vi "extract group name.vi"(9 "dictionary":T1, 10 "supported types":T2[](array[typedef]), 11 "TDMS datalogger configuration in":refnum<class "TDMS datalogger configuration.lvclass">) -> (2 "dictionary group names":T1)   [LabVIEW 2015, in "TDMS datalogger runtime.lvclass"]
uses:
  TDMS datalogger runtime.lvclass
  <vilib>/NI/Tag Bus/dictionary/full data dictionary.ctl
  <vilib>/NI/Tag Bus/tag/Data Type.ctl
  configuration/TDMS datalogger configuration.lvclass
  <vilib>/NI/Tag Bus/tag/tag descriptor.lvclass/tag descriptor.ctl
  <vilib>/NI/Tag Bus/tag/tag descriptor.lvclass
  <vilib>/NI/Tag Bus/dictionary/data dictionary.lvclass
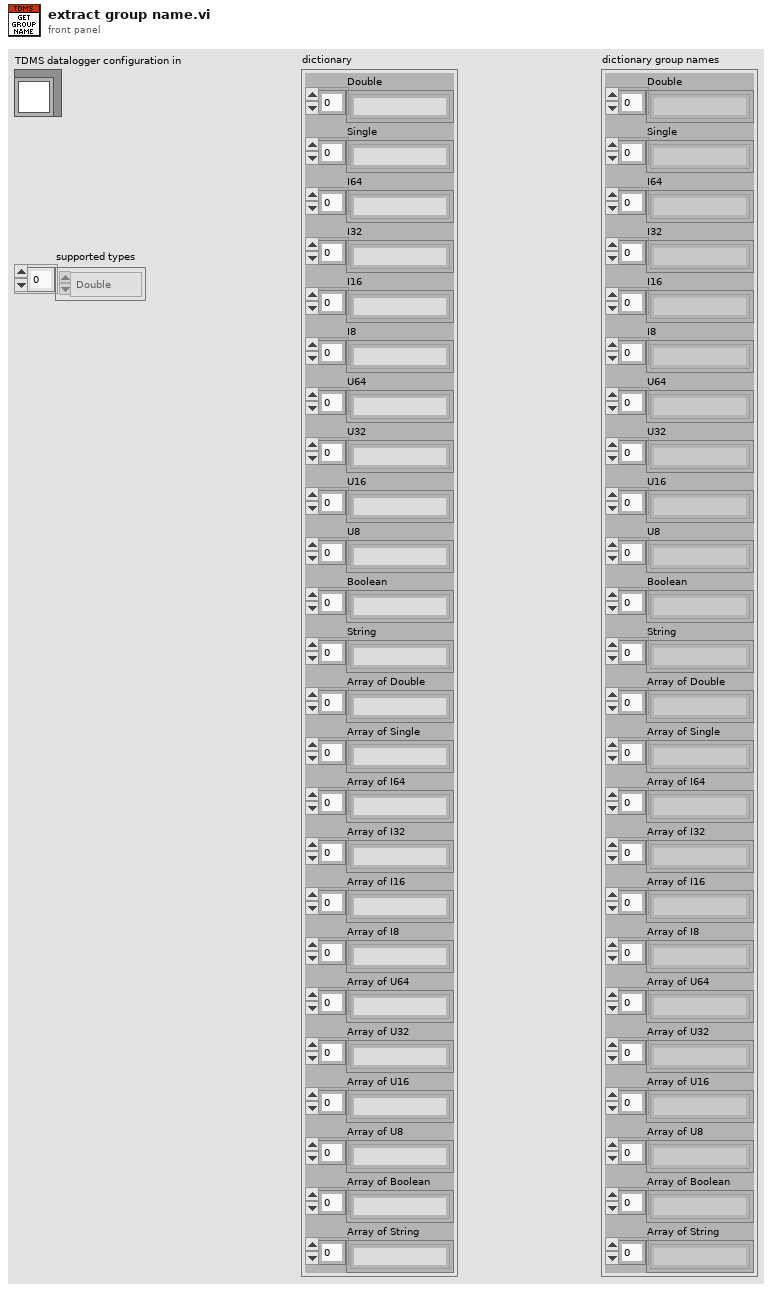
[diagram p1: front panel]
types:
  T1 = typedef "tag bus.lvlib/data dictionary.lvclass/full data dictionary.ctl" = cluster{"Double":string[], "Single":string[], "I64":string[], "I32":string[], "I16":string[], "I8":string[], "U64":string[], "U32":string[], "U16":string[], "U8":string[], "Boolean":string[], "String":string[], "Array of Double":string[], "Array of Single":string[], "Array of I64":string[], "Array of I32":string[], "Array of I16":string[], "Array of I8":string[], "Array of U64":string[], "Array of U32":string[], "Array of U16":string[], "Array of U8":string[], "Array of Boolean":string[], "Array of String":string[]}
  T2 = typedef "tag bus.lvlib/tag descriptor.lvclass/Data Type.ctl" = enum16{"Double", "Single", "I64", "I32", "I16", "I8", "U64", "U32", "U16", "U8", "Boolean", "String", "Array of Double", "Array of Single", "Array of I64", "Array of I32", "Array of I16", "Array of I8", "Array of U64", "Array of U32", "Array of U16", "Array of U8", "Array of Boolean", "Array of String"}
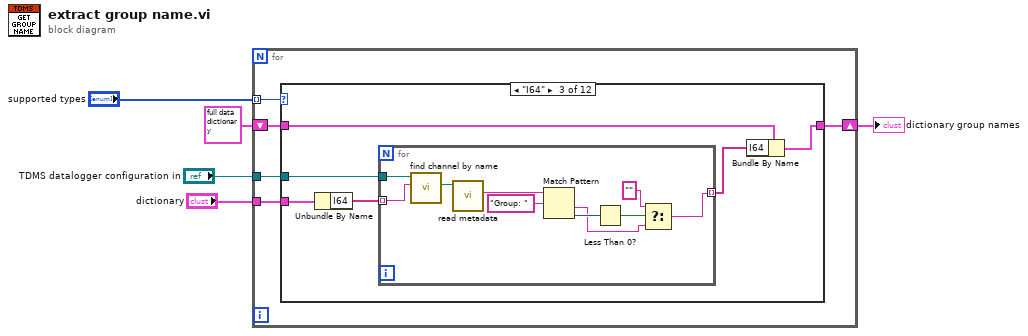
[diagram p0: block diagram]
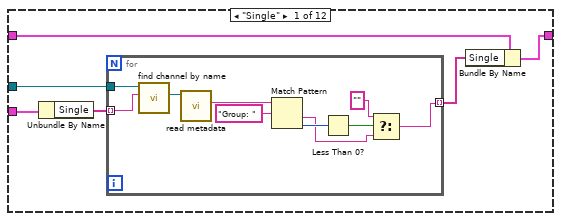
[diagram p2: hidden frame]
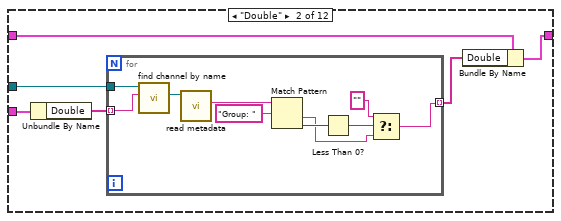
[diagram p3: hidden frame]
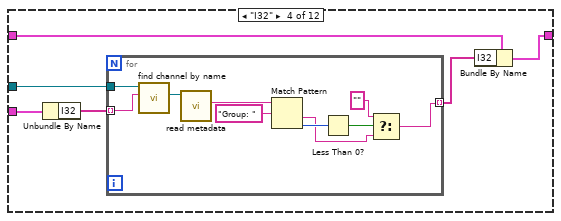
[diagram p4: hidden frame]
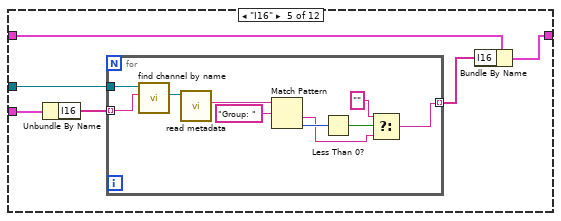
[diagram p5: hidden frame]
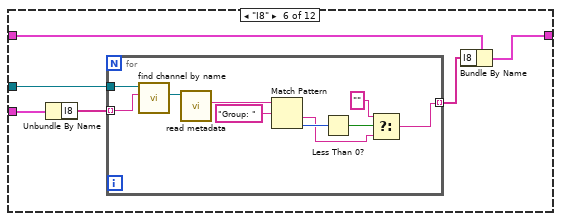
[diagram p6: hidden frame]
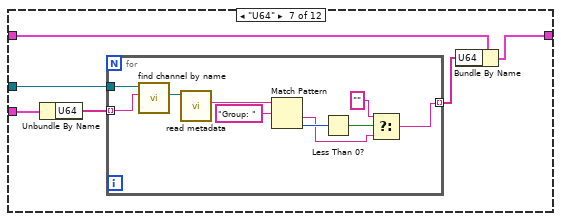
[diagram p7: hidden frame]
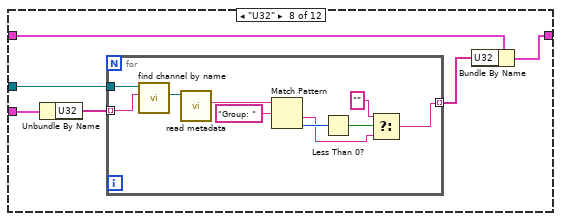
[diagram p8: hidden frame]
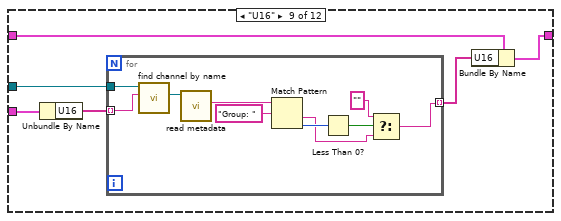
[diagram p9: hidden frame]
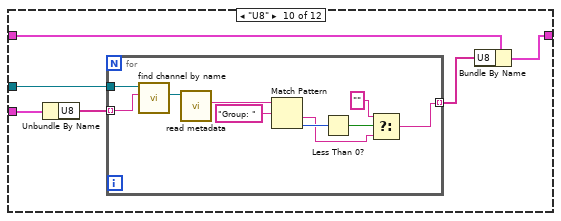
[diagram p10: hidden frame]
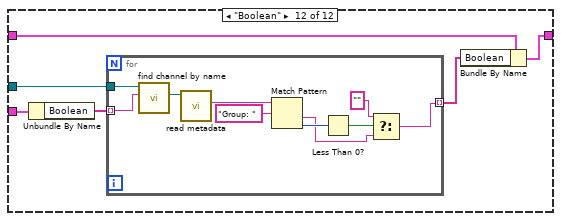
[diagram p12: hidden frame]
diagram:
  n1 = for {
    tunnel: "dictionary" -> [w9]
    tunnel: "supported types" -> [w10] mode=indexing
    tunnel: "TDMS datalogger configuration in" -> [w8]
    shift-right: [w6] -> w1
    shift-left: T1 {"Double"=[], "Single"=[], "I64"=[], "I32"=[], "I16"=[], "I8"=[], "U64"=[], "U32"=[], "U16"=[], "U8"=[], "Boolean"=[], "String"=[], "Array of Double"=[], "Array of Single"=[], "Array of I64"=[], "Array of I32"=[], "Array of I16"=[], "Array of I8"=[], "Array of U64"=[], "Array of U32"=[], "Array of U16"=[], "Array of U8"=[], "Array of Boolean"=[], "Array of String"=[]} ("dictionary metadata") -> [w7]
    n2 = case shown="\"Boolean\"" w10 {
      tunnel: w9 -> [w15 w32 w48 w64 w80 w96 w112 w128 w144 w160 _ w177]
      tunnel: w8 -> [w11 w28 w44 w59 w75 w92 w107 w124 w140 w156 _ w172]
      tunnel: w7 -> [w13 w30 w46 w63 w78 w95 w111 w127 w142 w158 w171 w175]
      tunnel: [w12 w31 w47 w62 w79 w94 w110 w126 w143 w159 w171 w176] -> w6
      frame "Single" {
        n3 = Unbundle By Name(w15) -> ("Single"=w14:string[])
        n4 = for {
          tunnel: w14 -> [w25] mode=indexing
          tunnel: [w19] -> w16 mode=indexing
          tunnel: w11 -> [w24]
          n5 = call "find channel by name.vi"("channel name"=w25, "TDMS datalogger configuration in"=w24) -> ("channel"=w26:refnum<class "TBM channel.lvclass">)  [unwired: 8 in, 1 out]
          n6 = call <vilib>:"read metadata.vi"("system tag in"=w26) -> ("metadata"=w23:string)  [unwired: 8 in, 2 out]
          n7 = Match Pattern(string=w23, regular expression="Group: ") -> (after substring=w18:string, offset past match=w21:i32)  [unwired: 1 in, 2 out]
          n8 = Less Than 0?(x=w21) -> (x < 0?=w20:bool)
          n9 = Select(t="", s=w20, f=w18) -> (s? t:f=w19:string)
        }
        n10 = Bundle By Name(cluster=w13, "Single"=w16) -> (w12:T1)
      }
      frame "Double" {
        n11 = Unbundle By Name(w32) -> ("Double"=w29:string[])
        n12 = for {
          tunnel: w29 -> [w41] mode=indexing
          tunnel: [w35] -> w27 mode=indexing
          tunnel: w28 -> [w40]
          n13 = call "find channel by name.vi"("channel name"=w41, "TDMS datalogger configuration in"=w40) -> ("channel"=w42:refnum<class "TBM channel.lvclass">)  [unwired: 8 in, 1 out]
          n14 = call <vilib>:"read metadata.vi"("system tag in"=w42) -> ("metadata"=w39:string)  [unwired: 8 in, 2 out]
          n15 = Match Pattern(string=w39, regular expression="Group: ") -> (after substring=w34:string, offset past match=w37:i32)  [unwired: 1 in, 2 out]
          n16 = Less Than 0?(x=w37) -> (x < 0?=w36:bool)
          n17 = Select(t="", s=w36, f=w34) -> (s? t:f=w35:string)
        }
        n18 = Bundle By Name(cluster=w30, "Double"=w27) -> (w31:T1)
      }
      frame "I64" {
        n19 = Unbundle By Name(w48) -> ("I64"=w45:string[])
        n20 = for {
          tunnel: w45 -> [w57] mode=indexing
          tunnel: [w51] -> w43 mode=indexing
          tunnel: w44 -> [w56]
          n21 = call "find channel by name.vi"("channel name"=w57, "TDMS datalogger configuration in"=w56) -> ("channel"=w58:refnum<class "TBM channel.lvclass">)  [unwired: 8 in, 1 out]
          n22 = call <vilib>:"read metadata.vi"("system tag in"=w58) -> ("metadata"=w55:string)  [unwired: 8 in, 2 out]
          n23 = Match Pattern(string=w55, regular expression="Group: ") -> (after substring=w50:string, offset past match=w53:i32)  [unwired: 1 in, 2 out]
          n24 = Less Than 0?(x=w53) -> (x < 0?=w52:bool)
          n25 = Select(t="", s=w52, f=w50) -> (s? t:f=w51:string)
        }
        n26 = Bundle By Name(cluster=w46, "I64"=w43) -> (w47:T1)
      }
      frame "I32" {
        n27 = Unbundle By Name(w64) -> ("I32"=w61:string[])
        n28 = for {
          tunnel: w61 -> [w73] mode=indexing
          tunnel: [w67] -> w60 mode=indexing
          tunnel: w59 -> [w72]
          n29 = call "find channel by name.vi"("channel name"=w73, "TDMS datalogger configuration in"=w72) -> ("channel"=w74:refnum<class "TBM channel.lvclass">)  [unwired: 8 in, 1 out]
          n30 = call <vilib>:"read metadata.vi"("system tag in"=w74) -> ("metadata"=w71:string)  [unwired: 8 in, 2 out]
          n31 = Match Pattern(string=w71, regular expression="Group: ") -> (after substring=w66:string, offset past match=w69:i32)  [unwired: 1 in, 2 out]
          n32 = Less Than 0?(x=w69) -> (x < 0?=w68:bool)
          n33 = Select(t="", s=w68, f=w66) -> (s? t:f=w67:string)
        }
        n34 = Bundle By Name(cluster=w63, "I32"=w60) -> (w62:T1)
      }
      frame "I16" {
        n35 = Unbundle By Name(w80) -> ("I16"=w77:string[])
        n36 = for {
          tunnel: w77 -> [w89] mode=indexing
          tunnel: [w83] -> w76 mode=indexing
          tunnel: w75 -> [w88]
          n37 = call "find channel by name.vi"("channel name"=w89, "TDMS datalogger configuration in"=w88) -> ("channel"=w90:refnum<class "TBM channel.lvclass">)  [unwired: 8 in, 1 out]
          n38 = call <vilib>:"read metadata.vi"("system tag in"=w90) -> ("metadata"=w87:string)  [unwired: 8 in, 2 out]
          n39 = Match Pattern(string=w87, regular expression="Group: ") -> (after substring=w82:string, offset past match=w85:i32)  [unwired: 1 in, 2 out]
          n40 = Less Than 0?(x=w85) -> (x < 0?=w84:bool)
          n41 = Select(t="", s=w84, f=w82) -> (s? t:f=w83:string)
        }
        n42 = Bundle By Name(cluster=w78, "I16"=w76) -> (w79:T1)
      }
      frame "I8" {
        n43 = Unbundle By Name(w96) -> ("I8"=w93:string[])
        n44 = for {
          tunnel: w93 -> [w105] mode=indexing
          tunnel: [w99] -> w91 mode=indexing
          tunnel: w92 -> [w104]
          n45 = call "find channel by name.vi"("channel name"=w105, "TDMS datalogger configuration in"=w104) -> ("channel"=w106:refnum<class "TBM channel.lvclass">)  [unwired: 8 in, 1 out]
          n46 = call <vilib>:"read metadata.vi"("system tag in"=w106) -> ("metadata"=w103:string)  [unwired: 8 in, 2 out]
          n47 = Match Pattern(string=w103, regular expression="Group: ") -> (after substring=w98:string, offset past match=w101:i32)  [unwired: 1 in, 2 out]
          n48 = Less Than 0?(x=w101) -> (x < 0?=w100:bool)
          n49 = Select(t="", s=w100, f=w98) -> (s? t:f=w99:string)
        }
        n50 = Bundle By Name(cluster=w95, "I8"=w91) -> (w94:T1)
      }
      frame "U64" {
        n51 = Unbundle By Name(w112) -> ("U64"=w109:string[])
        n52 = for {
          tunnel: w109 -> [w121] mode=indexing
          tunnel: [w115] -> w108 mode=indexing
          tunnel: w107 -> [w120]
          n53 = call "find channel by name.vi"("channel name"=w121, "TDMS datalogger configuration in"=w120) -> ("channel"=w122:refnum<class "TBM channel.lvclass">)  [unwired: 8 in, 1 out]
          n54 = call <vilib>:"read metadata.vi"("system tag in"=w122) -> ("metadata"=w119:string)  [unwired: 8 in, 2 out]
          n55 = Match Pattern(string=w119, regular expression="Group: ") -> (after substring=w114:string, offset past match=w117:i32)  [unwired: 1 in, 2 out]
          n56 = Less Than 0?(x=w117) -> (x < 0?=w116:bool)
          n57 = Select(t="", s=w116, f=w114) -> (s? t:f=w115:string)
        }
        n58 = Bundle By Name(cluster=w111, "U64"=w108) -> (w110:T1)
      }
      frame "U32" {
        n59 = Unbundle By Name(w128) -> ("U32"=w125:string[])
        n60 = for {
          tunnel: w125 -> [w137] mode=indexing
          tunnel: [w131] -> w123 mode=indexing
          tunnel: w124 -> [w136]
          n61 = call "find channel by name.vi"("channel name"=w137, "TDMS datalogger configuration in"=w136) -> ("channel"=w138:refnum<class "TBM channel.lvclass">)  [unwired: 8 in, 1 out]
          n62 = call <vilib>:"read metadata.vi"("system tag in"=w138) -> ("metadata"=w135:string)  [unwired: 8 in, 2 out]
          n63 = Match Pattern(string=w135, regular expression="Group: ") -> (after substring=w130:string, offset past match=w133:i32)  [unwired: 1 in, 2 out]
          n64 = Less Than 0?(x=w133) -> (x < 0?=w132:bool)
          n65 = Select(t="", s=w132, f=w130) -> (s? t:f=w131:string)
        }
        n66 = Bundle By Name(cluster=w127, "U32"=w123) -> (w126:T1)
      }
      frame "U16" {
        n67 = Unbundle By Name(w144) -> ("U16"=w141:string[])
        n68 = for {
          tunnel: w141 -> [w153] mode=indexing
          tunnel: [w147] -> w139 mode=indexing
          tunnel: w140 -> [w152]
          n69 = call "find channel by name.vi"("channel name"=w153, "TDMS datalogger configuration in"=w152) -> ("channel"=w154:refnum<class "TBM channel.lvclass">)  [unwired: 8 in, 1 out]
          n70 = call <vilib>:"read metadata.vi"("system tag in"=w154) -> ("metadata"=w151:string)  [unwired: 8 in, 2 out]
          n71 = Match Pattern(string=w151, regular expression="Group: ") -> (after substring=w146:string, offset past match=w149:i32)  [unwired: 1 in, 2 out]
          n72 = Less Than 0?(x=w149) -> (x < 0?=w148:bool)
          n73 = Select(t="", s=w148, f=w146) -> (s? t:f=w147:string)
        }
        n74 = Bundle By Name(cluster=w142, "U16"=w139) -> (w143:T1)
      }
      frame "U8" {
        n75 = Unbundle By Name(w160) -> ("U8"=w157:string[])
        n76 = for {
          tunnel: w157 -> [w169] mode=indexing
          tunnel: [w163] -> w155 mode=indexing
          tunnel: w156 -> [w168]
          n77 = call "find channel by name.vi"("channel name"=w169, "TDMS datalogger configuration in"=w168) -> ("channel"=w170:refnum<class "TBM channel.lvclass">)  [unwired: 8 in, 1 out]
          n78 = call <vilib>:"read metadata.vi"("system tag in"=w170) -> ("metadata"=w167:string)  [unwired: 8 in, 2 out]
          n79 = Match Pattern(string=w167, regular expression="Group: ") -> (after substring=w162:string, offset past match=w165:i32)  [unwired: 1 in, 2 out]
          n80 = Less Than 0?(x=w165) -> (x < 0?=w164:bool)
          n81 = Select(t="", s=w164, f=w162) -> (s? t:f=w163:string)
        }
        n82 = Bundle By Name(cluster=w158, "U8"=w155) -> (w159:T1)
      }
      frame Default {
      }
      frame "Boolean" {
        n83 = Unbundle By Name(w177) -> ("Boolean"=w174:string[])
        n84 = for {
          tunnel: w174 -> [w186] mode=indexing
          tunnel: [w180] -> w173 mode=indexing
          tunnel: w172 -> [w185]
          n85 = call "find channel by name.vi"("channel name"=w186, "TDMS datalogger configuration in"=w185) -> ("channel"=w187:refnum<class "TBM channel.lvclass">)  [unwired: 8 in, 1 out]
          n86 = call <vilib>:"read metadata.vi"("system tag in"=w187) -> ("metadata"=w184:string)  [unwired: 8 in, 2 out]
          n87 = Match Pattern(string=w184, regular expression="Group: ") -> (after substring=w179:string, offset past match=w182:i32)  [unwired: 1 in, 2 out]
          n88 = Less Than 0?(x=w182) -> (x < 0?=w181:bool)
          n89 = Select(t="", s=w181, f=w179) -> (s? t:f=w180:string)
        }
        n90 = Bundle By Name(cluster=w175, "Boolean"=w173) -> (w176:T1)
      }
    }
  }
  "dictionary group names" <- w1
